vi "2-10.vi"(1 "input_decimals":T2, 2 "input_minors":T2) -> (0 "output":T1)   [LabVIEW 2013]
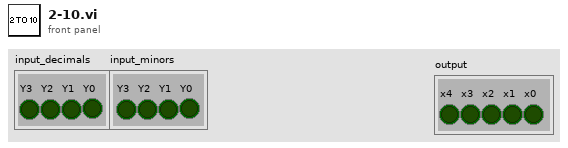
[diagram p1: front panel]
types:
  T1 = cluster{"x4":bool, "x3":bool, "x2":bool, "x1":bool, "x0":bool}
  T2 = cluster{"Y3":bool, "Y2":bool, "Y1":bool, "Y0":bool}
  T3 = cluster{"Y0":bool, "Y3":bool, "Y2":bool, "Y1":bool, "Y0":bool}
  T4 = cluster{"y4":bool, "y3":bool, "y2":bool, "y1":bool, "y0":bool}
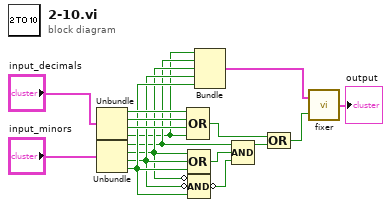
[diagram p0: block diagram]
diagram:
  n1 = Unbundle("input_decimals") -> ("Y3"=w13:bool, "Y2"=w12:bool, "Y1"=w11:bool, "Y0"=w4:bool)
  n2 = Unbundle("input_minors") -> ("Y3"=w5:bool, "Y2"=w6:bool, "Y1"=w7:bool, "Y0"=w8:bool)
  n3 = Compound Arithmetic op=OR(w13, w12, w11, w4) -> (w9:bool)
  n4 = Compound Arithmetic op=OR(w6, w7, w8) -> (w15:bool)
  n5 = Compound Arithmetic op=AND(invert w6, invert w7, w8) -> (invert w14:bool)
  n6 = Bundle("Y0"=w4, "Y3"=w5, "Y2"=w6, "Y1"=w7, "Y0"=w8) -> (w3:T3)  [unwired: 1 in]
  n7 = Compound Arithmetic op=AND(w5, w15, w14) -> (w10:bool)
  n8 = Compound Arithmetic op=OR(w9, w10) -> (w1:bool)
  n9 = call "fixer.vi"("2-10 flag"=w1, "input"=w3) -> ("output"=→"output":T4)
